vi "Get triangular number series.vi"(8 "error in (no error)":errorcluster, 11 "n = generate this many terms (dflt=100)":u32=100) -> (0 "error out":errorcluster, 3 "Triangular numbers":u64[](array[numeric]))   [LabVIEW 2021, in "Numeric Utilities.lvlib"]
uses:
  Numeric Utilities.lvlib
panel:
  # "Development\ncontrols/indicators useful for development and testing, but which are not outputs of the VI"
  # "Input\nInputs to the VI"
  # "Output\nOutputs of the VI"
  # "Description\n\nBlank VI with error handling case. \n\nSummarize the use of this VI in this space."
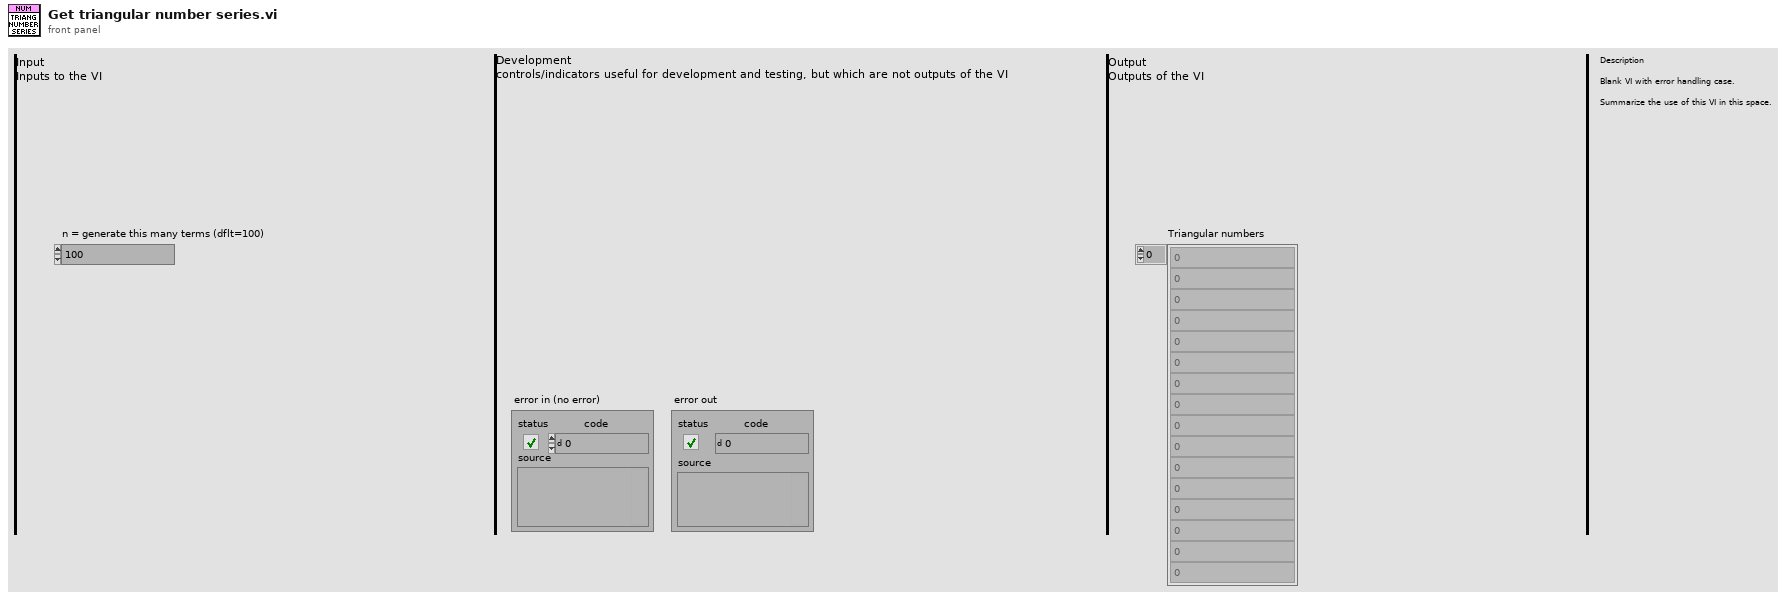
[diagram p1: front panel]
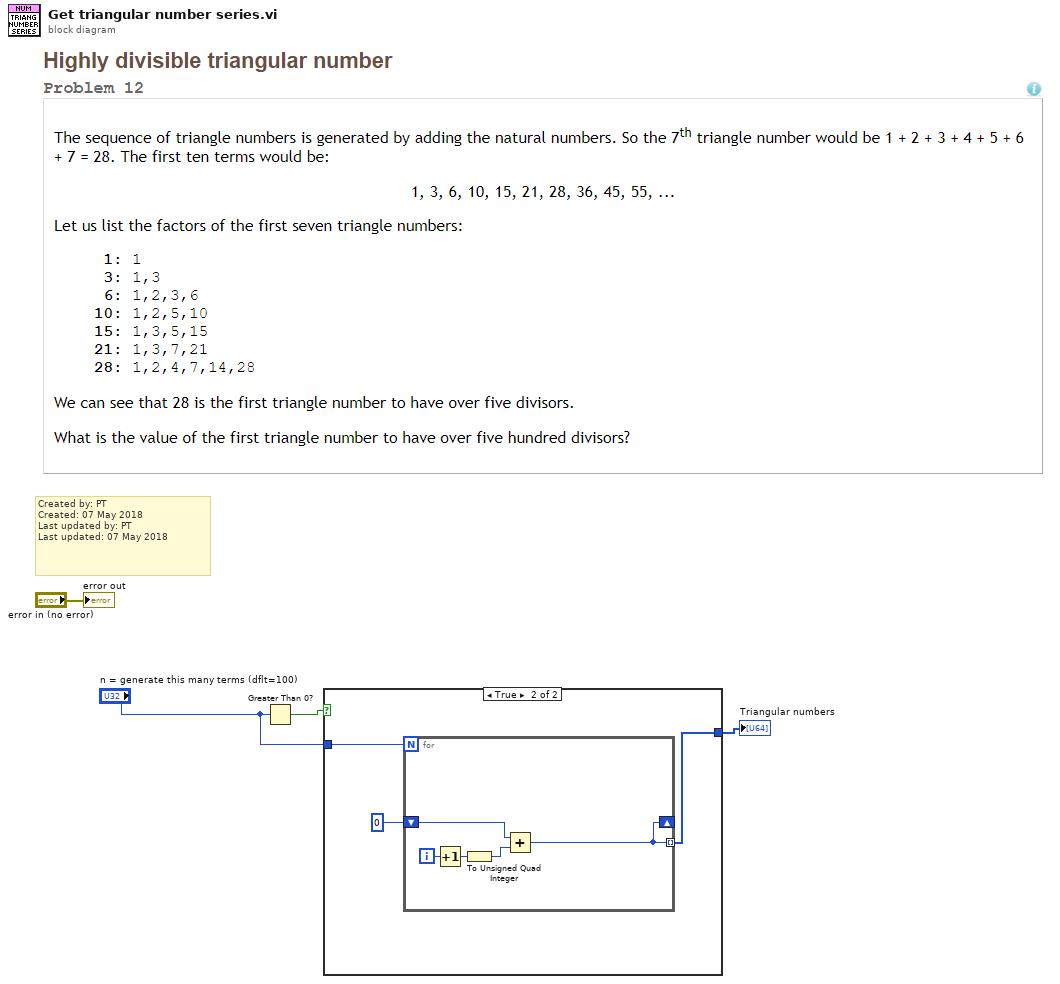
[diagram p0: block diagram]
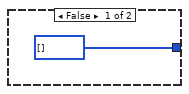
[diagram p2: hidden frame]
diagram:
  # "Created by: PT\nCreated: 07 May 2018\nLast updated by: PT\nLast updated: 07 May 2018"
  n1 = Greater Than 0?(x="n = generate this many terms (dflt=100)") -> (x > 0?=w3:bool)
  n2 = case shown="True" w3 {
    tunnel: [u64[] [] ("Triangular numbers") w6] -> w2
    tunnel: "n = generate this many terms (dflt=100)" -> [_ w8]
    frame False {
    }
    frame True {
      n3 = for {
        N: w8 -> [_]
        shift-right: [w10] -> _
        shift-left: u64 0 -> [w13]
        tunnel: [w10] -> w6 mode=indexing
        i -> [w12]
        n4 = Increment(x=w12) -> (x+1=w9:i32)
        n5 = To Unsigned Quad Integer(1:w9) -> (0:w11:u64)
        n6 = Add(x=w13, y=w11) -> (x+y=w10:u64)
      }
    }
  }
  "Triangular numbers" <- w2
  "error out" <- "error in (no error)"
